vi "ACT_Limit_Setpoint.vi"(8 "error in":errorcluster, 10 "3 JSA10 FT112 XQ75":dbl, 11 "SI750.lvclass":refnum<class "SI750.lvclass">) -> (0 "error out":errorcluster, 2 "ACT Setpoint":dbl, 3 "SI750.lvclass out":refnum<class "SI750.lvclass">)   [LabVIEW 2022 SP3, in "SI750.lvclass"]
uses:
  SI750.lvclass
  SI750.lvclass/SI750.ctl
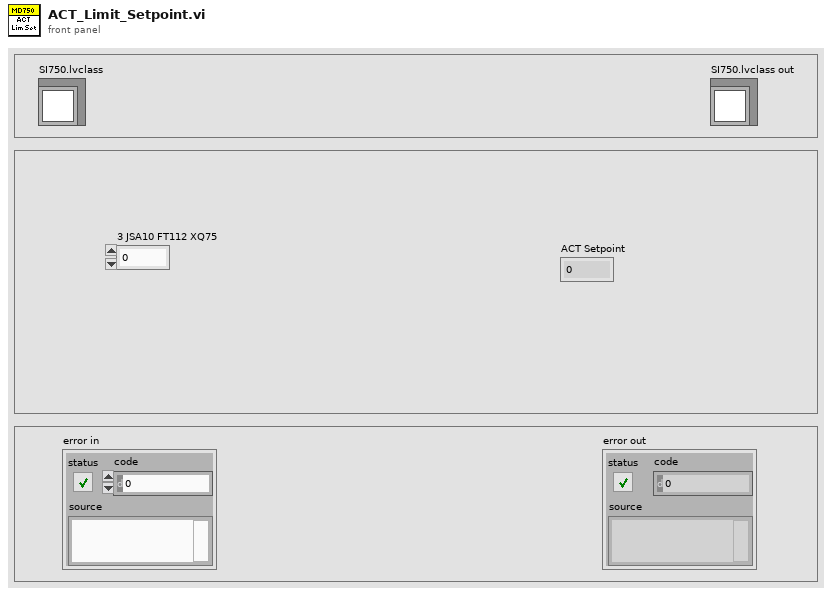
[diagram p1: front panel]
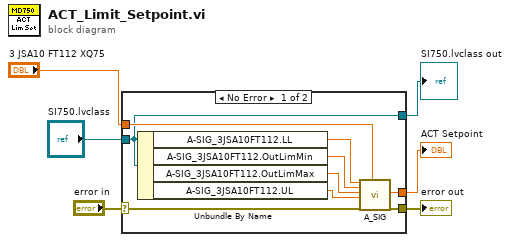
[diagram p0: block diagram]
diagram:
  n1 = case shown="No Error" "error in" {
    selector: "error in" -> [w10 w17]
    tunnel: "3 JSA10 FT112 XQ75" -> [w15 _]
    tunnel: "SI750.lvclass" -> [w7 w16]
    tunnel: [w9 w17] -> w2
    tunnel: [w8 _] -> w3
    tunnel: [w7 w16] -> w1
    frame No Error {
      n2 = Unbundle By Name(w7) -> ("A-SIG_3JSA10FT112.LL"=w14:dbl, "A-SIG_3JSA10FT112.OutLimMin"=w13:dbl, "A-SIG_3JSA10FT112.OutLimMax"=w12:dbl, "A-SIG_3JSA10FT112.UL"=w11:dbl)
      n3 = call "A_SIG.vi"("LL"=w14, "OutLimMin"=w13, "OutLimMax"=w12, "UL"=w11, "error in (no error)"=w10, "Input"=w15) -> ("A_SIG_out"=w8:dbl, "error out"=w9:errorcluster)  [unwired: 12 in]
    }
    frame Error {
    }
  }
  "ACT Setpoint" <- w3
  "error out" <- w2
  "SI750.lvclass out" <- w1
